vi "WT1800 Close Instruments.vi"(0 "WT1800 Instruments In":refnum<visa-resource-name>[](array[refnum]), 7 "Buffer Complete In":bool, 11 "error in":errorcluster, 12 "DSA Errors In":errorcluster) -> (4 "WT1800 Instruments Out":refnum<visa-resource-name>[](array[refnum]), 13 "Buffer Complete Out":bool, 15 "error out":errorcluster)   [LabVIEW 2021]
uses:
  <instrlib>/Yokogawa WT1800 Series/Yokogawa WT1800 Series.lvlib
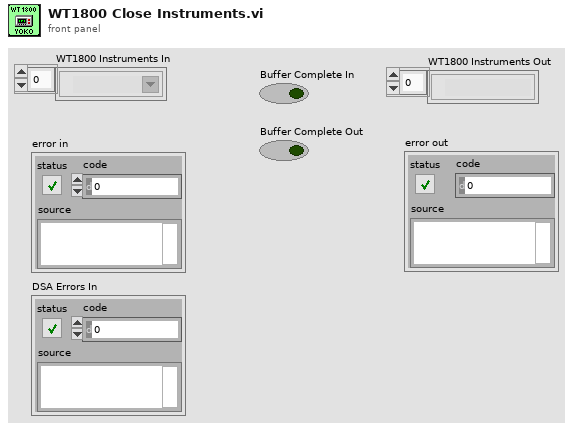
[diagram p1: front panel]
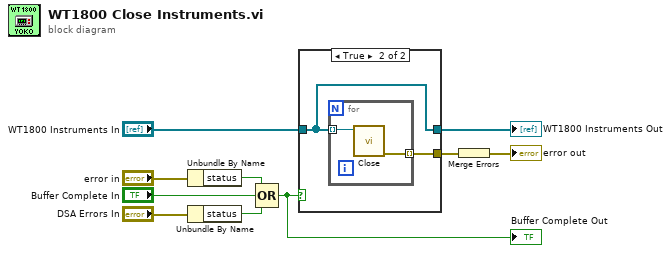
[diagram p0: block diagram]
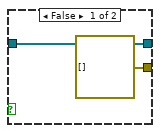
[diagram p2: hidden frame]
diagram:
  n1 = Unbundle By Name("error in") -> ("status"=w7:bool)
  n2 = Unbundle By Name("DSA Errors In") -> ("status"=w6:bool)
  n3 = Compound Arithmetic op=OR(w7, "Buffer Complete In", w6) -> (w5:bool)
  "Buffer Complete Out" <- w5
  n4 = case shown="True" w5 {
    tunnel: [errorcluster[] [] w14] -> w2
    tunnel: "WT1800 Instruments In" -> [w12 w13]
    tunnel: [w12 w13] -> w9
    frame False {
    }
    frame True {
      n5 = for {
        tunnel: [w16] -> w14 mode=indexing
        tunnel: w13 -> [w15] mode=indexing
        n6 = call <instrlib>:"Close.vi"("VISA resource name"=w15) -> ("error out"=w16:errorcluster)  [unwired: 10 in]
      }
    }
  }
  "WT1800 Instruments Out" <- w9
  n7 = Merge Errors(w2) -> (→"error out":errorcluster)
